vi "Load_Comparitor_Cluster.vi"() -> ()   [LabVIEW 2015]
uses:
  ADAM_Comparitor.ctl
  Anemometry/Anemometry Sub Vis/Globals/Constants_global.vi
  ADAM_Global.vi
panel:
  out "Channel Values Out":string[][](array[string])
  out "Ch names Out":string[](array[string])
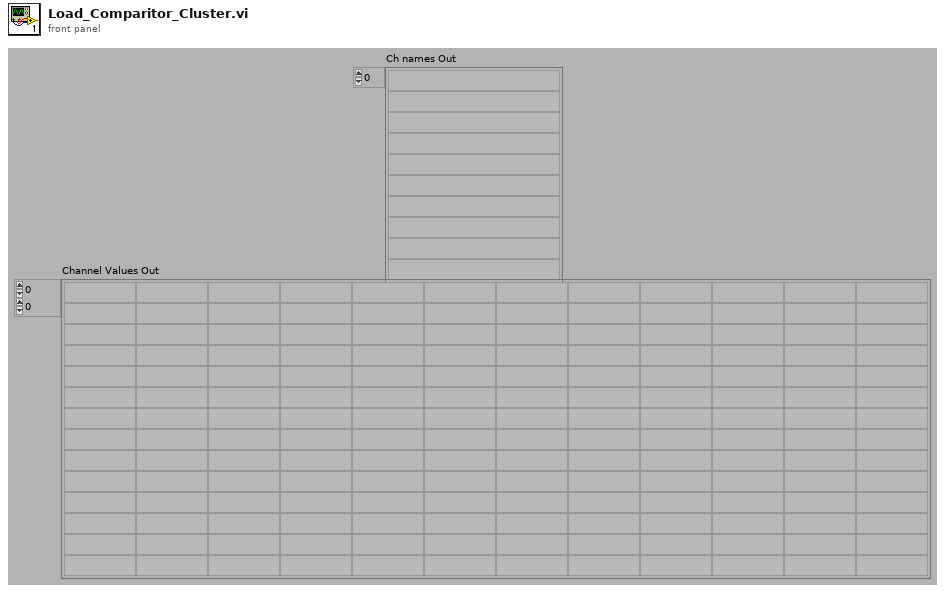
[diagram p1: front panel]
types:
  T1 = typedef "ADAM_Comparitor.ctl" = cluster{"Ch to Monitor":string, "Channels to Kill":string, "Warn if Above":dbl, "Warn if Below":dbl, "Kill if Above":dbl, "Kill if Below":dbl, "Hysteresis Margin":dbl, "Averaging TIme (s)":dbl, "Warn Status":bool, "Kill Status":bool, "Extra Email addresses":string}
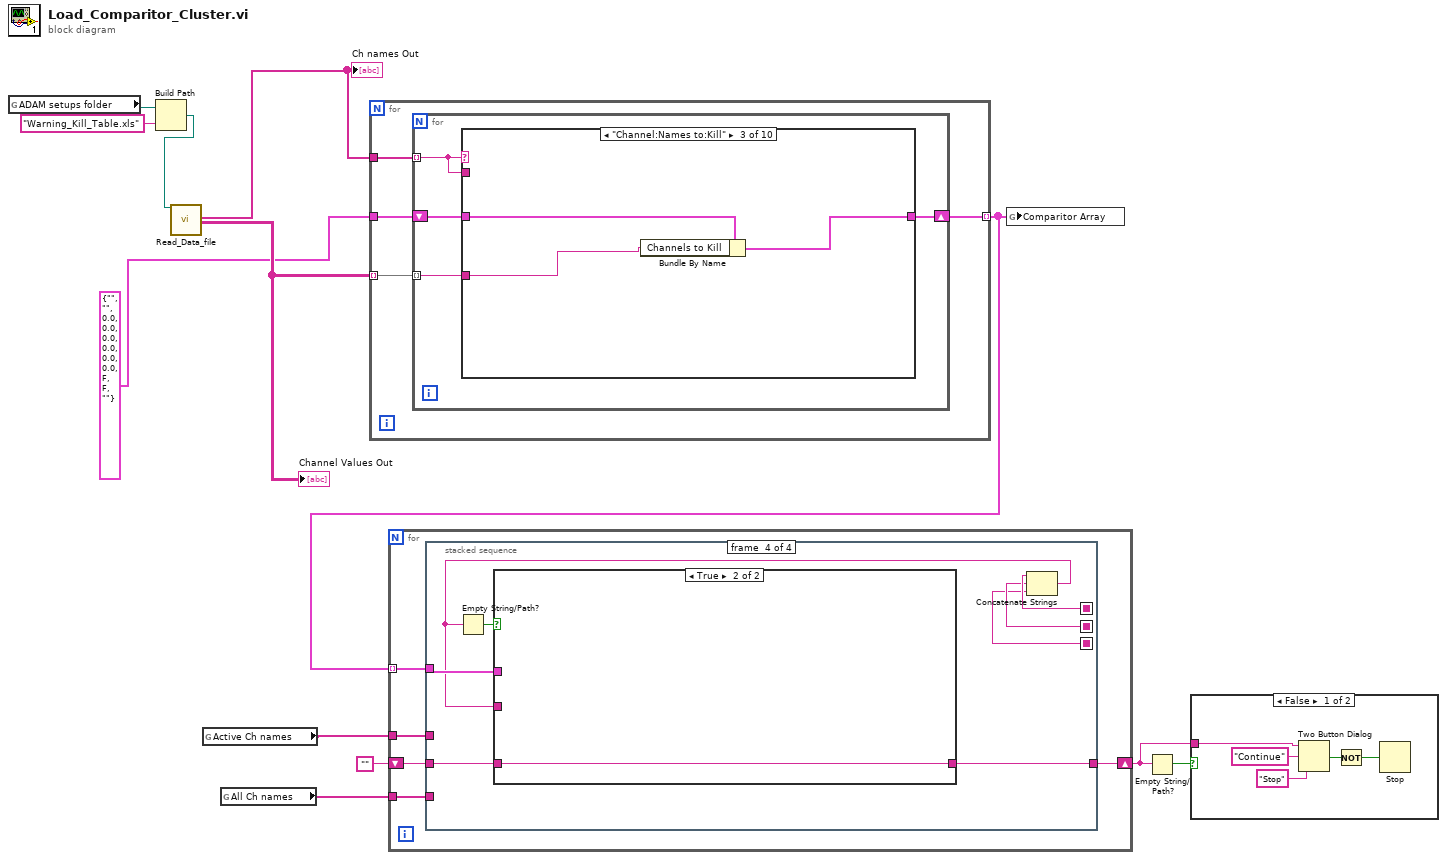
[diagram p0: block diagram]
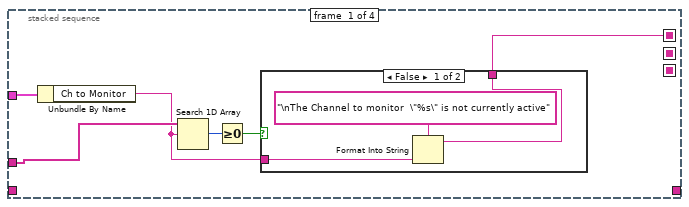
[diagram p3: hidden frame]
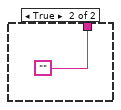
[diagram p4: hidden frame]
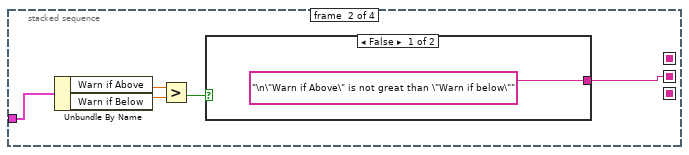
[diagram p5: hidden frame]
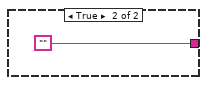
[diagram p6: hidden frame]
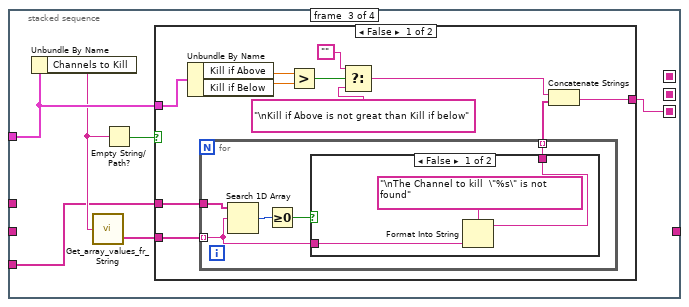
[diagram p7: hidden frame]
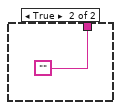
[diagram p8: hidden frame]
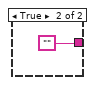
[diagram p9: hidden frame]
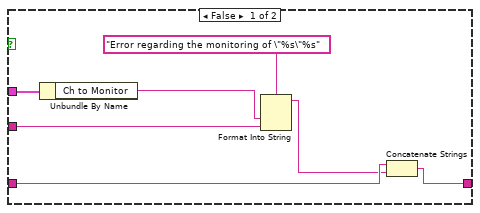
[diagram p10: hidden frame]
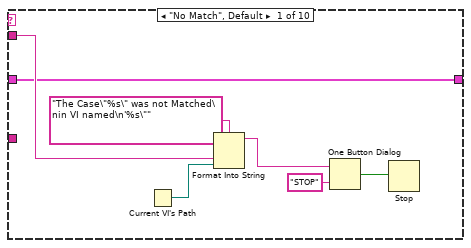
[diagram p11: hidden frame]
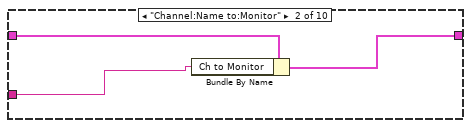
[diagram p12: hidden frame]
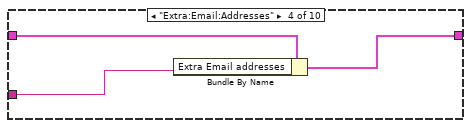
[diagram p13: hidden frame]
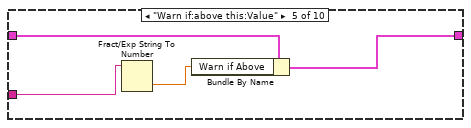
[diagram p14: hidden frame]
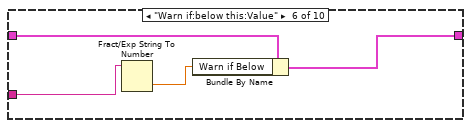
[diagram p15: hidden frame]
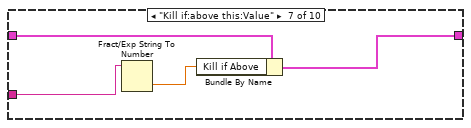
[diagram p16: hidden frame]
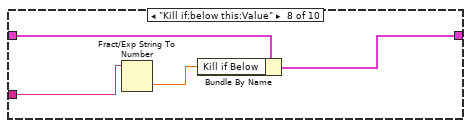
[diagram p17: hidden frame]
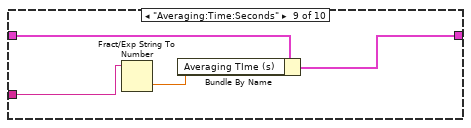
[diagram p18: hidden frame]
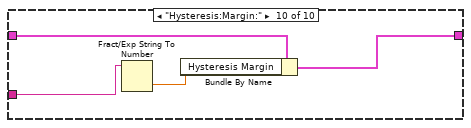
[diagram p19: hidden frame]
diagram:
  n1 = global read "Constants_global.vi" "ADAM setups folder"() -> (w5:path)
  n2 = Build Path(base path=w5, name or relative path="Warning_Kill_Table.xls") -> (appended path=w3:path)
  n3 = call "Read_Data_file.vi"("Results file"=w3) -> ("Ch names Out"=w12:string[], "Channel Values Out"=w11:string[][])  [unwired: 9 in, 8 out]
  "Ch names Out" <- w12
  "Channel Values Out" <- w11
  n4 = global read "ADAM_Global.vi" "Active Ch names"() -> (w2:string[])
  n5 = global read "ADAM_Global.vi" "All Ch names"() -> (w1:string[])
  n6 = for {
    tunnel: w12 -> [w16]
    tunnel: w11 -> [w15] mode=indexing
    tunnel: T1 {"Ch to Monitor"="", "Channels to Kill"="", "Warn if Above"=0.0, "Warn if Below"=0.0, "Kill if Above"=0.0, "Kill if Below"=0.0, "Hysteresis Margin"=0.0, "Averaging TIme (s)"=0.0, "Warn Status"=FALSE, "Kill Status"=FALSE, "Extra Email addresses"=""} ("Cluster") -> [w14]
    tunnel: [w13] -> w9 mode=indexing
    n7 = for {
      tunnel: w16 -> [w17] mode=indexing
      shift-right: [w19] -> w13
      shift-left: w14 -> [w18]
      tunnel: w15 -> [w20] mode=indexing
      n8 = case shown="\"Channel:Names to:Kill\"" w17 {
        tunnel: w20 -> [_ w30 w33 w36 w38 w42 w46 w50 w54 w58]
        tunnel: [w21 w29 w32 w35 w40 w44 w48 w52 w56 w60] -> w19
        tunnel: w18 -> [w21 w28 w31 w34 w39 w43 w47 w51 w55 w59]
        tunnel: w17 -> [w22 _ _ _ _ _ _ _ _ _]
        frame "No Match", Default {
          n9 = Current VI's Path() -> (path=w23:path)
          n10 = Format Into String(format string="The Case\"%s\" was not Matched\nin VI named\n'%s\"" ("Format String"), w22, w23) -> (resulting string=w26:string)  [unwired: 2 in, 1 out]
          n11 = One Button Dialog(message=w26, button name ("OK")="STOP") -> (true=w24:bool)
          n12 = Stop(stop? (T)=w24) -> ()
        }
        frame "Channel:Name to:Monitor" {
          n13 = Bundle By Name(cluster=w28, "Ch to Monitor"=w30) -> (w29:T1)
        }
        frame "Channel:Names to:Kill" {
          n14 = Bundle By Name(cluster=w31, "Channels to Kill"=w33) -> (w32:T1)
        }
        frame "Extra:Email:Addresses" {
          n15 = Bundle By Name(cluster=w34, "Extra Email addresses"=w36) -> (w35:T1)
        }
        frame "Warn if:above this:Value" {
          n16 = Fract/Exp String To Number(string=w38) -> (number=w37:dbl)  [unwired: 3 in, 1 out]
          n17 = Bundle By Name(cluster=w39, "Warn if Above"=w37) -> (w40:T1)
        }
        frame "Warn if:below this:Value" {
          n18 = Fract/Exp String To Number(string=w42) -> (number=w41:dbl)  [unwired: 3 in, 1 out]
          n19 = Bundle By Name(cluster=w43, "Warn if Below"=w41) -> (w44:T1)
        }
        frame "Kill if:above this:Value" {
          n20 = Fract/Exp String To Number(string=w46) -> (number=w45:dbl)  [unwired: 3 in, 1 out]
          n21 = Bundle By Name(cluster=w47, "Kill if Above"=w45) -> (w48:T1)
        }
        frame "Kill if:below this:Value" {
          n22 = Fract/Exp String To Number(string=w50) -> (number=w49:dbl)  [unwired: 3 in, 1 out]
          n23 = Bundle By Name(cluster=w51, "Kill if Below"=w49) -> (w52:T1)
        }
        frame "Averaging:Time:Seconds" {
          n24 = Fract/Exp String To Number(string=w54) -> (number=w53:dbl)  [unwired: 3 in, 1 out]
          n25 = Bundle By Name(cluster=w55, "Averaging TIme (s)"=w53) -> (w56:T1)
        }
        frame "Hysteresis:Margin:" {
          n26 = Fract/Exp String To Number(string=w58) -> (number=w57:dbl)  [unwired: 3 in, 1 out]
          n27 = Bundle By Name(cluster=w59, "Hysteresis Margin"=w57) -> (w60:T1)
        }
      }
    }
  }
  n28 = for {
    tunnel: w9 -> [w65] mode=indexing
    shift-right: [w62] -> w6
    shift-left: "" -> [w63]
    tunnel: w2 -> [w64]
    tunnel: w1 -> [w61]
    n29 = stacked-sequence {
      seq-local: [_ w80 _ _] -> [_ _ _ w116]
      seq-local: [_ _ w86 _] -> [_ _ _ w115]
      seq-local: [w66 _ _ _] -> [_ _ _ w117]
      tunnel: w65 -> [w70 w76 w87 w113]
      tunnel: w64 -> [w69 _ _ _]
      tunnel: w63 -> [_ _ _ w111]
      tunnel: [_ _ _ w110] -> w62
      tunnel: w61 -> [_ _ w83 _]
      frame #0 {
        n30 = Unbundle By Name(w70) -> ("Ch to Monitor"=w67:string)
        n31 = Search 1D Array(1D array=w69, element=w67) -> (index of element=w68:i32)  [unwired: 1 in]
        n32 = Greater Or Equal To 0?(x=w68) -> (x >= 0?=w71:bool)
        n33 = case shown="False" w71 {
          tunnel: w67 -> [w74 _]
          tunnel: [w72 ""] -> w66
          frame False {
            n34 = Format Into String(format string="\nThe Channel to monitor  \"%s\" is not currently active", w74) -> (resulting string=w72:string)  [unwired: 2 in, 1 out]
          }
          frame True {
          }
        }
      }
      frame #1 {
        n35 = Unbundle By Name(w76) -> ("Warn if Above"=w79:dbl, "Warn if Below"=w78:dbl)
        n36 = Greater?(x=w79, y=w78) -> (0:w77:bool)
        n37 = case shown="False" w77 {
          tunnel: ["\n\"Warn if Above\" is not great than \"Warn if below\"" ""] -> w80
          frame False {
          }
          frame True {
          }
        }
      }
      frame #2 {
        n38 = Unbundle By Name(w87) -> ("Channels to Kill"=w85:string)
        n39 = call "Get_array_values_fr_String.vi"("String Value"=w85) -> ("String array"=w84:string[])  [unwired: 1 out]
        n40 = Empty String/Path?(string/path=w85) -> (empty?=w88:bool)
        n41 = case shown="False" w88 {
          tunnel: w87 -> [w99 _]
          tunnel: [w90 ""] -> w86
          tunnel: w83 -> [w96 _]
          tunnel: w84 -> [w89 _]
          frame False {
            n42 = Unbundle By Name(w99) -> ("Kill if Above"=w98:dbl, "Kill if Below"=w97:dbl)
            n43 = for {
              tunnel: w96 -> [w104]
              tunnel: [w101] -> w92 mode=indexing
              tunnel: w89 -> [w100] mode=indexing
              n44 = Search 1D Array(1D array=w104, element=w100) -> (index of element=w103:i32)  [unwired: 1 in]
              n45 = Greater Or Equal To 0?(x=w103) -> (x >= 0?=w102:bool)
              n46 = case shown="False" w102 {
                tunnel: w100 -> [w107 _]
                tunnel: [w105 ""] -> w101
                frame False {
                  n47 = Format Into String(format string="\nThe Channel to kill  \"%s\" is not found", w107) -> (resulting string=w105:string)  [unwired: 2 in, 1 out]
                }
                frame True {
                }
              }
            }
            n48 = Greater?(x=w98, y=w97) -> (0:w95:bool)
            n49 = Select(t="", s=w95, f="\nKill if Above is not great than Kill if below") -> (s? t:f=w91:string)
            n50 = Concatenate Strings(w91, w92) -> (w90:string)
          }
          frame True {
          }
        }
      }
      frame #3 {
        n51 = Concatenate Strings(w117, w116, w115) -> (w112:string)
        n52 = Empty String/Path?(string/path=w112) -> (empty?=w114:bool)
        n53 = case shown="True" w114 {
          tunnel: w113 -> [w124 _]
          tunnel: w112 -> [w121 _]
          tunnel: w111 -> [w120 w125]
          tunnel: [w118 w125] -> w110
          frame False {
            n54 = Unbundle By Name(w124) -> ("Ch to Monitor"=w123:string)
            n55 = Format Into String(format string="Error regarding the monitoring of \"%s\"%s", w123, w121) -> (resulting string=w119:string)  [unwired: 2 in, 1 out]
            n56 = Concatenate Strings(w120, w119) -> (w118:string)
          }
          frame True {
          }
        }
      }
    }
  }
  n57 = global write "ADAM_Global.vi" "Comparitor Array"(w9) -> ()
  n58 = Empty String/Path?(string/path=w6) -> (empty?=w7:bool)
  n59 = case shown="False" w7 {
    tunnel: w6 -> [w126 _]
    frame False {
      n60 = Two Button Dialog(message=w126, 1:"Stop" ("F button name (\"Cancel\")"), 2:"Continue" ("T button name (\"OK\")")) -> (T button?=w128:bool)
      n61 = Not(x=w128) -> (.not. x?=w127:bool)
      n62 = Stop(stop? (T)=w127) -> ()
    }
    frame True {
    }
  }
